vi "OTF_subtraction_triple.vi"(0 "Buffer Length":i32, 1 "Max Triggers":i32, 5 "Buffer":u32[](array[numeric]), 7 "Triggers In":u64, 9 "Expected Delay":dbl, 11 "Max Delay":dbl, 12 "ofl":u64) -> (3 "ofl out":u64, 4 "Event Data":dbl[][](array[numeric]), 6 "Coincidence Delays":dbl[](array[numeric]), 8 "Coincidences":u32, 10 "Triggers":u64, 14 "Delays":dbl[](array[numeric]), 15 "Shifted Delays":dbl[](array[numeric]))   [LabVIEW 2023]
panel:
  out "Trues":dbl
  out "Coincidence Triggers":u64
  out "Time":dbl[](array[numeric])
  out "Channel":u64[](array[numeric])
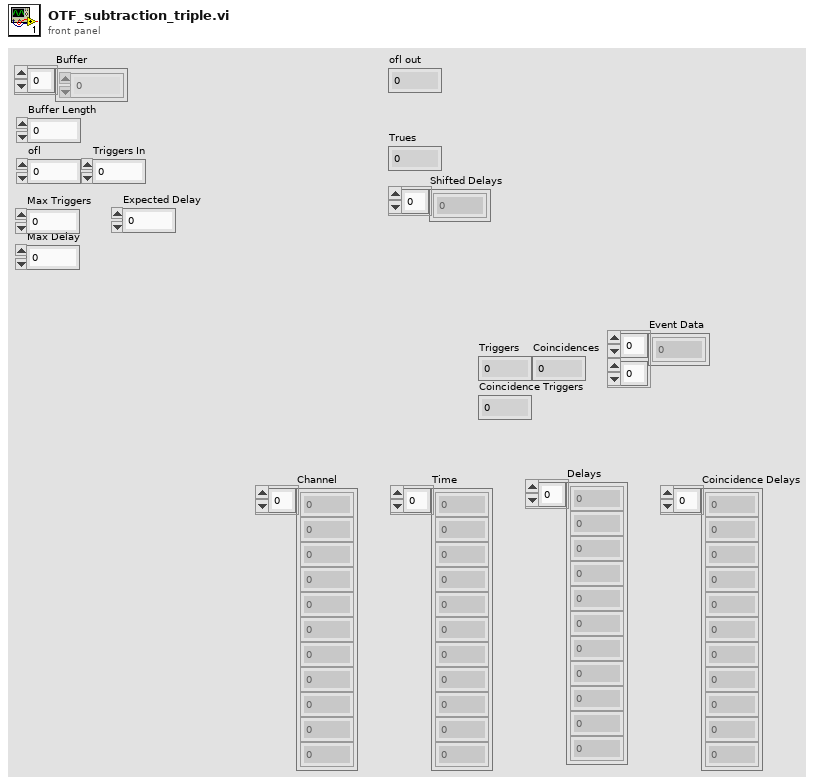
[diagram p1: front panel]
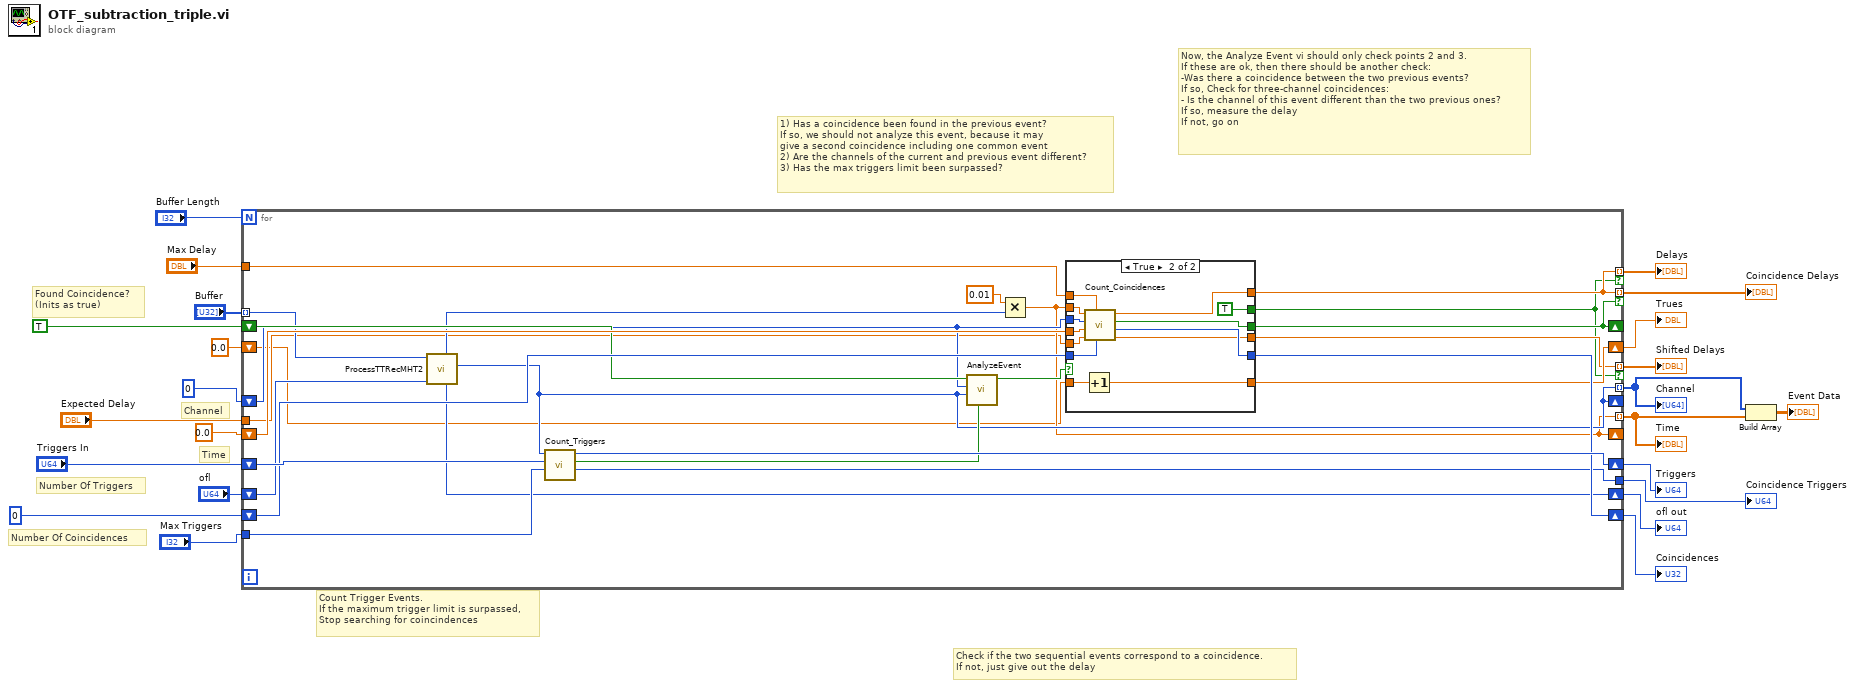
[diagram p0: block diagram]
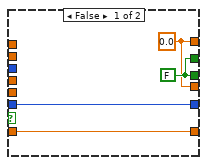
[diagram p2: hidden frame]
diagram:
  # "Now, the Analyze Event vi should only check points 2 and 3.\nIf these are ok, then there should be another check:\n-Was there a coincidence between the two previous events?\nIf so, Check for three-channel coincidences:\n- Is the channel of this event different than the two previous ones?\nIf so, measure the delay\nIf not, go on"
  # "Check if the two sequential events correspond to a coincidence. \nIf not, just give out the delay"
  # "Count Trigger Events.\nIf the maximum trigger limit is surpassed,\nStop searching for coincindences"
  # "1) Has a coincidence been found in the previous event? \nIf so, we should not analyze this event, because it may\ngive a second coincidence including one common event\n2) Are the channels of the current and previous event different?\n3) Has the max triggers limit been surpassed?"
  # "Found Coincidence?\n(Inits as true)"
  # "Time"
  # "Channel"
  # "Number Of Coincidences"
  # "Number Of Triggers"
  n1 = for {
    N: "Buffer Length" -> [_]
    shift-right: [w30] -> _
    shift-left: 0.0 ("number: 0 to 1") -> [w46]
    tunnel: [w37] -> w19 mode=indexing if=w25
    shift-right: [w35] -> _
    shift-left: u32 0 ("number") -> [w38]
    tunnel: [w35] -> w8 mode=indexing
    tunnel: [w30] -> w7 mode=indexing
    shift-right: [w48] -> w23
    shift-left: "Triggers In" -> [w49]
    tunnel: [w37] -> w5 mode=indexing if=w36
    shift-right: [w45] -> w17
    shift-left: u32 0 -> [w47]
    shift-right: [w36] -> _
    shift-left: TRUE ("Is Coincidence?") -> [w43]
    tunnel: [w42] -> w15
    tunnel: "Max Triggers" -> [w40]
    tunnel: "Max Delay" -> [w39]
    tunnel: "Buffer" -> [w34] mode=indexing
    shift-right: [w32] -> w9
    shift-left: "ofl" -> [w33]
    tunnel: "Expected Delay" -> [w28]
    shift-right: [w27] -> w2
    shift-left: 0.0 -> [w24]
    tunnel: [w26] -> w1 mode=indexing if=w25
    n2 = call "ProcessTTRecMHT2.vi"("oflcorr_in"=w33, "rawbits"=w34) -> ("channel"=w35:u32, "oflcorr_out"=w32:u64, "timetag"=w31:u64)  [unwired: 4 in, 3 out]
    n3 = call "Count_Triggers.vi"("Max Triggers"=w40, "Triggers In"=w49, "channel"=w35) -> ("Coincidence Triggers"=w42:u64, "Max triggers?"=w41:bool, "Total Triggers Out"=w48:u64)  [unwired: 6 in]
    n4 = call "AnalyzeEvent.vi"("Max triggers?"=w41, "Channel - Current"=w35, "Channel - Previous"=w38, 11:w43) -> ("Analyze?"=w44:bool)  [unwired: 7 in]
    n5 = Multiply(x=0.01, y=w31) -> (x*y=w30:dbl)
    n6 = case shown="True" w44 {
      tunnel: w47 -> [w53 w66]
      tunnel: w39 -> [_ w65]
      tunnel: w46 -> [_ w64]
      tunnel: w38 -> [_ w63]
      tunnel: w30 -> [_ w62]
      tunnel: [w52 w61] -> w36
      tunnel: [w50 w60] -> w37
      tunnel: [w53 w59] -> w45
      tunnel: [w52 TRUE ("Is Coincidence?")] -> w25
      tunnel: w28 -> [_ w57]
      tunnel: w24 -> [w51 w56]
      tunnel: [w51 w55] -> w27
      tunnel: [w50 w54] -> w26
      frame False {
        w50 = 0.0 ("Delay")
        w52 = FALSE ("Is Coincidence?")
      }
      frame True {
        n7 = Increment(x=w56) -> (x+1=w55:dbl)
        n8 = call "Count_Coincidences.vi"("Coincidences In"=w66, "Max Delay"=w65, "Expected Delay"=w57, "Time - Previous"=w64, "Channel-Previous"=w63, "Time-Current"=w62) -> ("Shifted Delay"=w54:dbl, "Coincidences Out"=w59:u32, "Is Coincidence?"=w61:bool, "Delay"=w60:dbl)  [unwired: 2 in]
      }
    }
  }
  "Delays" <- w19
  "Channel" <- w8
  "Time" <- w7
  "Triggers" <- w23
  "Coincidences" <- w17
  "Coincidence Delays" <- w5
  "Coincidence Triggers" <- w15
  "ofl out" <- w9
  "Trues" <- w2
  "Shifted Delays" <- w1
  n9 = Build Array(w8, w7) -> (→"Event Data":dbl[][])
